vi "GenericRamp.vi"() -> ()   [LabVIEW 2016]
panel:
  in  "Digital ramp destination":enum32{"Frequency", "Phase", "Amplitude"}(ring)=enum."Amplitude"
  in  "frequency Hz (0..400M)":dbl=1000000.0 format="%^#_6e"
  in  "Ramp type":enum32{"Frequency", "Phase", "Amplitude"}(ring)=enum."Amplitude"
  out "Step seperation (us)":dbl=0.4
  in  "Ramp duration (us)":dbl=40.0 format="%#_6f"
  in  "Ramp trigger source":T1(ring)=enum."BNC_IN_A_RISING"
  in  "Step Size":dbl=0.01 format="%#_6f"
  in  "Max Value":dbl=1.0 format="%#_13g"
  in  "Min Value":dbl format="%#_6f"
  in  "Channels":T2(ring)=enum."Channel 1"
  out "return count":u32=378
  out "error out":errorcluster={"status"=TRUE, "code"=-1073807339, "source"="VISA Read in GenericRamp.vi"}
  out "read buffer":string
  out "Final instruction string":string="dds 1 reset\rdcp 1 spi:CFR2=0x1020080\rdcp 1 spi:STP0=0x418937\rdcp 1 wait:0h:\rdcp 1 update:u\rdcp 1 spi:DRL=0xFFFC000000000000\rdcp 1 spi:DRSS=0x28F5C29028F5C29\rdcp 1 spi:DRR=0x640064\rdcp 1 spi:CFR2=0x280080\rdcp 1 wait::BNC_IN_A_RISING\rdcp 1 update:u+d\rdcp 1 wait:12500h:\rdcp 1 update:-d\rdcp 1 spi:CFR2=0x1000080\rdcp 1 spi:STP0=0x418937\rdcp 1 wait:5000h:\rdcp 1 update:u\rdcp 1 start\r"
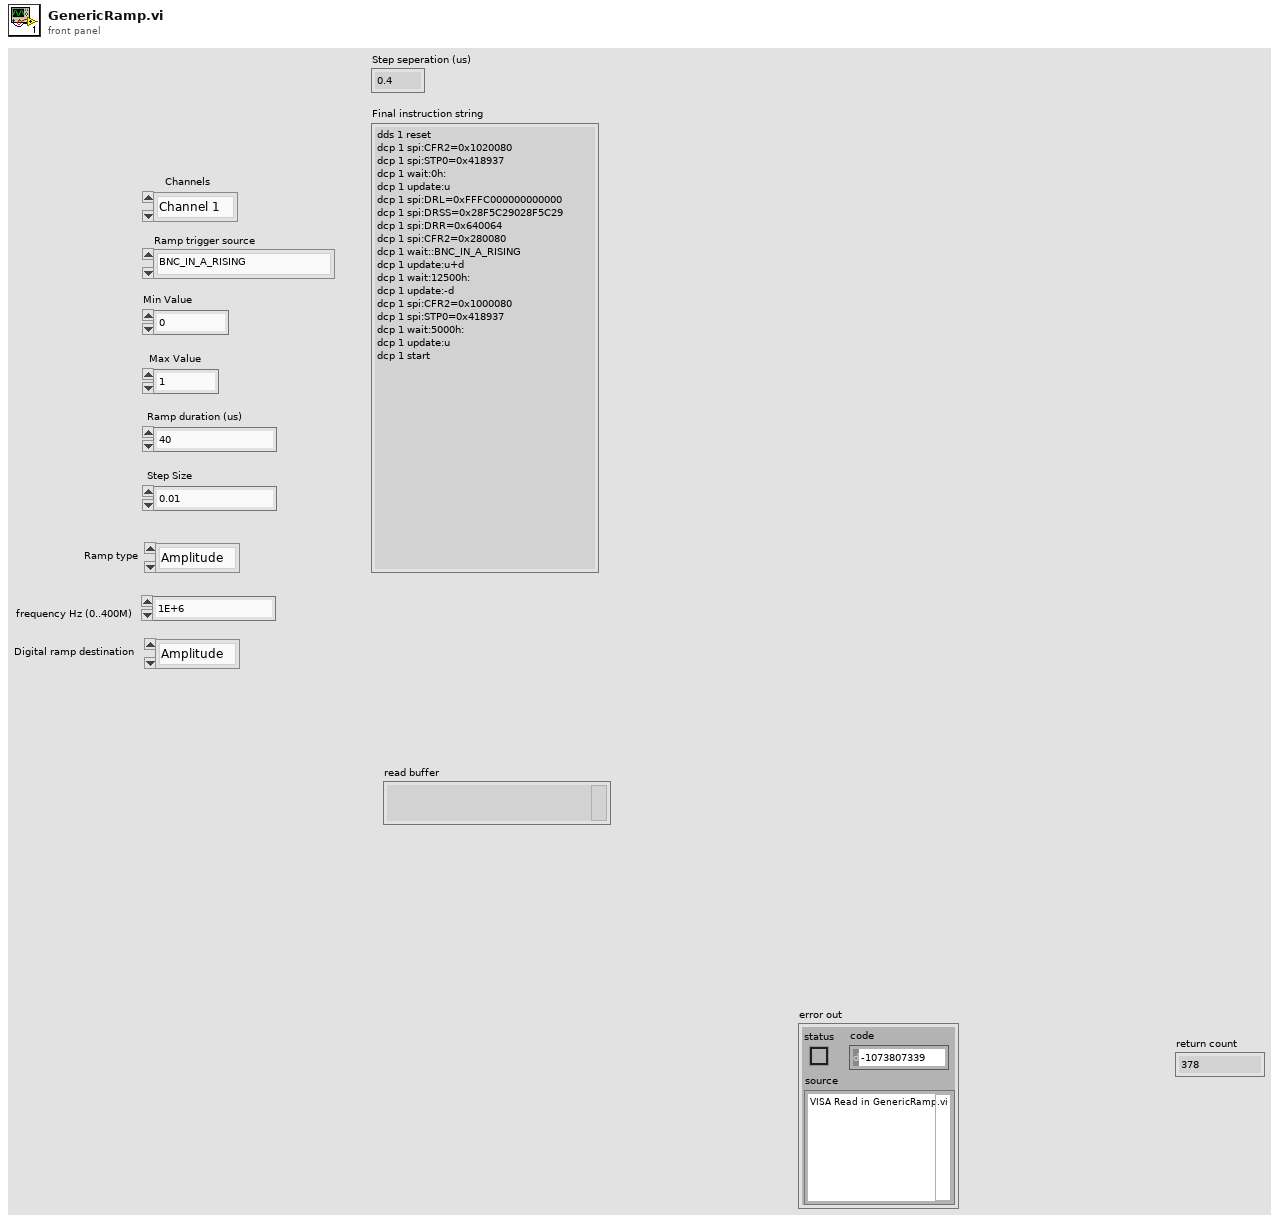
[diagram p1: front panel]
types:
  T1 = enum32{"O_RAMP_SWP_OVR", "RAM_SWP_OVR", "O_DROVER", "DROVER", "O_SPI_FIFO_EV1", "SPI_FIFO_EV1", "O_SPI_FIFO_EV0", "SPI_FIFO_EV0", "O_SPI_FIFO_FLUSHED", "SPI_FIFO_FLUSHED", "BNC_IN_B_LEVEL", "BNC_IN_B_FALLING", "BNC_IN_B_RISING", "BNC_IN_A_LEVEL", "BNC_IN_A_FALLING", "BNC_IN_A_RISING", "ALL_SPI_FIFOS_FLUSHED", "NONE"}
  T2 = enum32{"Channel 0", "Channel 1", "Both channels"}
  T3 = cluster{"Enable ASF from STP (F)":bool, "Digital ramp enable (F)":bool, "Digital ramp no-dwell high (F)":bool, "Digital ramp no-dwell low (F)":bool, "Matched latency enable (T)":bool, "Parallel data port enable (F)":bool}
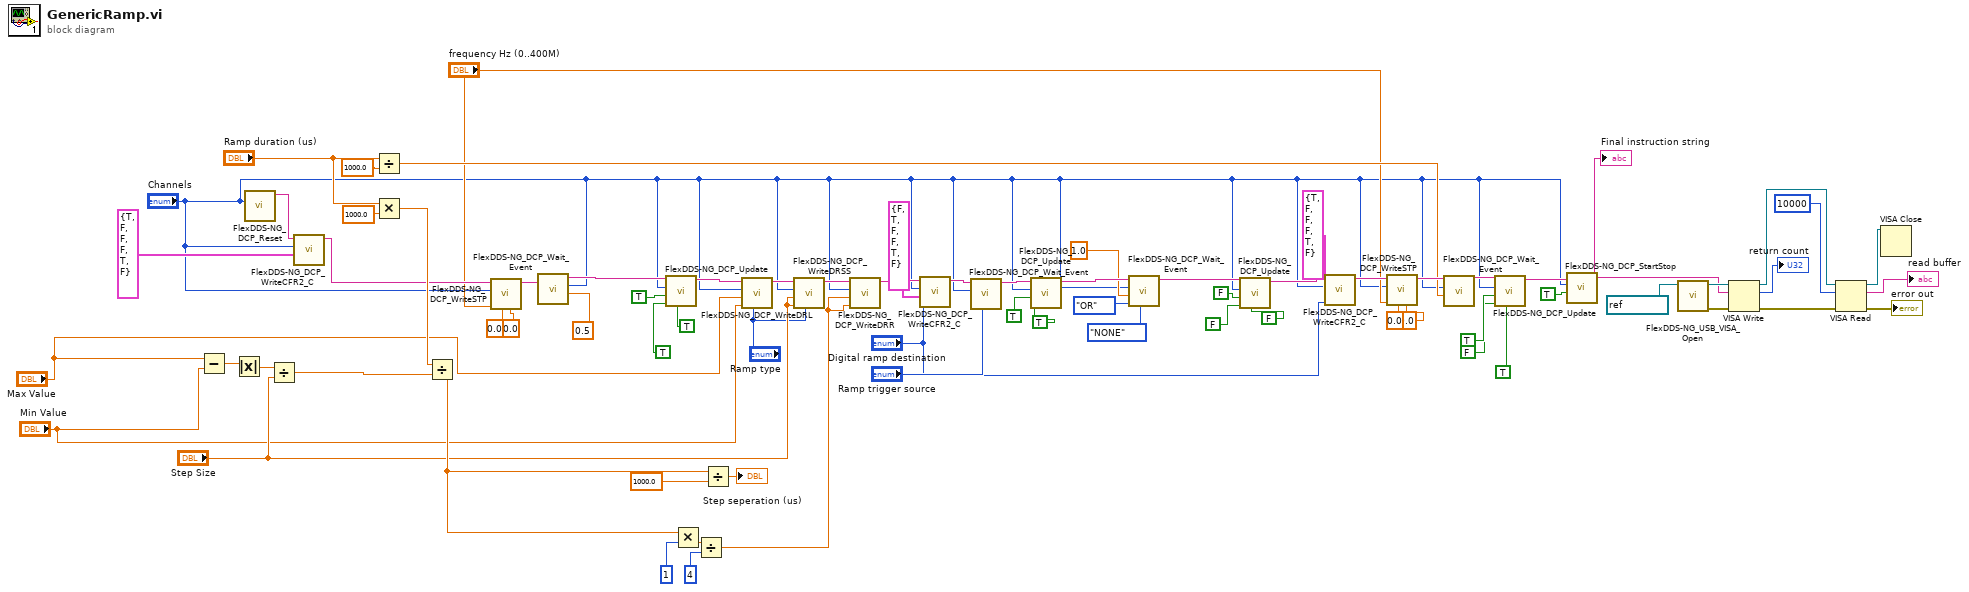
[diagram p0: block diagram]
diagram:
  n1 = Subtract(x="Max Value", y="Min Value") -> (x-y=w7:dbl)
  n2 = Absolute Value(x=w7) -> (abs(x)=w6:dbl)
  n3 = call "FlexDDS-NG_DCP_Reset.vi"("Channels"="Channels") -> ("appended instruction string"=w26:string)  [unwired: 10 in]
  n4 = Divide(x=w6, y="Step Size") -> (x/y=w37:dbl)
  n5 = call "FlexDDS-NG_DCP_WriteCFR2_C.vi"("CFR2 bits"=T3 {"Enable ASF from STP (F)"=TRUE, "Digital ramp enable (F)"=FALSE, "Digital ramp no-dwell high (F)"=FALSE, "Digital ramp no-dwell low (F)"=FALSE, "Matched latency enable (T)"=TRUE, "Parallel data port enable (F)"=FALSE} ("CFR2 bits 2"), "Channels"="Channels", "initial instruction string"=w26) -> ("appended instruction string"=w27:string)  [unwired: 8 in]
  n6 = Divide(x="Ramp duration (us)", y=1000.0) -> (x/y=w11:dbl)
  n7 = Multiply(x="Ramp duration (us)", y=1000.0) -> (x*y=w36:dbl)
  n8 = Divide(x=w36, y=w37) -> (x/y=w35:dbl)
  n9 = call "FlexDDS-NG_DCP_WriteSTP.vi"("phase degrees (0..360)"=0.0, "amplitude (0..1)"=0.0, "frequency Hz (0..400M)"="frequency Hz (0..400M)", "Channels"="Channels", "initial instruction string"=w27) -> ("appended instruction string"=w2:string)  [unwired: 6 in]
  n10 = call "FlexDDS-NG_DCP_Wait_Event.vi"("waiting time [ms]"=0.5, "Channels in"="Channels", "appended instruction string in"=w2) -> ("appended instruction string"=w21:string)  [unwired: 8 in]
  n11 = call "FlexDDS-NG_DCP_Update.vi"("ONLY IO_UPDATE"=TRUE, "DRCTL(true=+, false=-)"=TRUE ("DRCTL(true=+, false=-) 2"), "IO_UPDATE(true=u, false = '')"=TRUE ("IO_UPDATE(true=u, false = '')  2"), "Channels"="Channels", "appended instruction string in"=w21) -> ("appended instruction string out"=w20:string)  [unwired: 6 in]
  n12 = Multiply(x=w35, y=u16 1) -> (x*y=w40:dbl)
  n13 = Divide(x=w40, y=u16 4) -> (x/y=w1:dbl)
  n14 = Divide(x=w35, y=1000.0 ("x/y")) -> (x/y=→"Step seperation (us)":dbl)
  n15 = call "FlexDDS-NG_DCP_WriteDRL.vi"("Ramp type"="Ramp type", "low limit"="Min Value", "high limit"="Max Value", "Channels"="Channels", "initial instruction string"=w20) -> ("appended instruction string"=w64:string)  [unwired: 6 in]
  n16 = call "FlexDDS-NG_DCP_WriteDRSS.vi"("Ramp type"="Ramp type", "increment step size"="Step Size", "decrement step size"="Step Size", "Channels"="Channels", "initial instruction string"=w64) -> ("appended instruction string"=w63:string)  [unwired: 6 in]
  n17 = call "FlexDDS-NG_DCP_WriteDRR.vi"("digital ramp positive slope rate"=w1, "digital ramp negative slope rate"=w1, "Channels"="Channels", "initial instruction string"=w63) -> ("appended instruction string"=w62:string)  [unwired: 7 in]
  n18 = call "FlexDDS-NG_DCP_WriteCFR2_C.vi"("Digital ramp destination"="Digital ramp destination", "CFR2 bits"=T3 {"Enable ASF from STP (F)"=FALSE, "Digital ramp enable (F)"=TRUE, "Digital ramp no-dwell high (F)"=FALSE, "Digital ramp no-dwell low (F)"=FALSE, "Matched latency enable (T)"=TRUE, "Parallel data port enable (F)"=FALSE}, "Channels"="Channels", "initial instruction string"=w62) -> ("appended instruction string"=w57:string)  [unwired: 7 in]
  n19 = call "FlexDDS-NG_DCP_Wait_Event.vi"("Event 1"="Ramp trigger source", "Channels in"="Channels", "appended instruction string in"=w57) -> ("appended instruction string"=w56:string)  [unwired: 8 in]
  n20 = call "FlexDDS-NG_DCP_Update.vi"("DRCTL(true=+, false=-)"=TRUE, "IO_UPDATE(true=u, false = '')"=TRUE, "Channels"="Channels", "appended instruction string in"=w56) -> ("appended instruction string out"=w51:string)  [unwired: 7 in]
  n21 = call "FlexDDS-NG_DCP_Wait_Event.vi"("Event 1"=T1."NONE", "AND/OR"=enum32{"AND", "OR"}."OR", "waiting time [ms]"=1.0 ("y"), "Channels in"="Channels", "appended instruction string in"=w51) -> ("appended instruction string"=w13:string)  [unwired: 6 in]
  n22 = call "FlexDDS-NG_DCP_Update.vi"("ONLY IO_UPDATE"=FALSE, "DRCTL(true=+, false=-)"=FALSE ("DRCTL(true=+, false=-) 2"), "IO_UPDATE(true=u, false = '')"=FALSE ("IO_UPDATE(true=u, false = '')  2"), "Channels"="Channels", "appended instruction string in"=w13) -> ("appended instruction string out"=w14:string)  [unwired: 6 in]
  n23 = call "FlexDDS-NG_DCP_WriteCFR2_C.vi"("Digital ramp destination"="Digital ramp destination", "CFR2 bits"=T3 {"Enable ASF from STP (F)"=TRUE, "Digital ramp enable (F)"=FALSE, "Digital ramp no-dwell high (F)"=FALSE, "Digital ramp no-dwell low (F)"=FALSE, "Matched latency enable (T)"=TRUE, "Parallel data port enable (F)"=FALSE}, "Channels"="Channels", "initial instruction string"=w14) -> ("appended instruction string"=w44:string)  [unwired: 7 in]
  n24 = call "FlexDDS-NG_DCP_WriteSTP.vi"("phase degrees (0..360)"=0.0, "amplitude (0..1)"=0.0, "frequency Hz (0..400M)"="frequency Hz (0..400M)", "Channels"="Channels", "initial instruction string"=w44) -> ("appended instruction string"=w43:string)  [unwired: 6 in]
  n25 = call "FlexDDS-NG_DCP_Wait_Event.vi"("waiting time [ms]"=w11, "Channels in"="Channels", "appended instruction string in"=w43) -> ("appended instruction string"=w42:string)  [unwired: 8 in]
  n26 = call "FlexDDS-NG_DCP_Update.vi"("ONLY IO_UPDATE"=TRUE, "DRCTL(true=+, false=-)"=FALSE ("DRCTL(true=+, false=-) 2"), "IO_UPDATE(true=u, false = '')"=TRUE ("IO_UPDATE(true=u, false = '')  2"), "Channels"="Channels", "appended instruction string in"=w42) -> ("appended instruction string out"=w47:string)  [unwired: 6 in]
  n27 = call "FlexDDS-NG_DCP_StartStop.vi"("start (T) stop (F)"=TRUE, "Channels"="Channels", "initial instruction string"=w47) -> ("appended instruction string"=w19:string)  [unwired: 8 in]
  "Final instruction string" <- w19
  n28 = call "FlexDDS-NG_USB_VISA_Open.vi"("FlexDDS-NG USB VISA resource name (COM)"=refnum<visa-resource-name> "COM7") -> ("error out"=w66:errorcluster, "FlexDDS-NG USB VISA resource name out"=w67:refnum<visa-resource-name>)  [unwired: 9 in]
  n29 = VISA Write(VISA resource name=w67, write buffer=w19, error in (no error)=w66) -> (VISA resource name out=w71:refnum<visa-resource-name>, return count=→"return count":u32, error out=w69:errorcluster)
  n30 = VISA Read(VISA resource name=w71, byte count=u32 10000, error in (no error)=w69) -> (VISA resource name out=w74:refnum<visa-resource-name>, read buffer=→"read buffer":string, error out=→"error out":errorcluster)  [unwired: 1 out]
  n31 = VISA Close(VISA resource name=w74) -> ()  [unwired: 1 in, 1 out]
